vi "GetGyroAngle.vi"(8 "error in":errorcluster) -> (0 "error out":errorcluster, 3 "Angle":dbl)   [LabVIEW 2016]
uses:
  Robot Global Data.vi
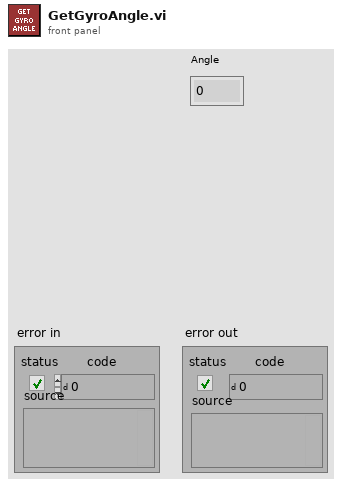
[diagram p1: front panel]
types:
  T1 = cluster{"Yaw":dbl, "Roll":dbl, "Pitch":dbl, "Heading":dbl, "Fused Heading":dbl}
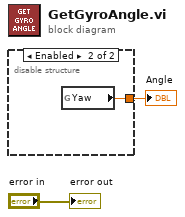
[diagram p0: block diagram]
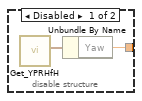
[diagram p2: hidden frame]
diagram:
  n1 = disable-structure shown="Enabled" {
    disable-tunnel: [w3 w5] -> w1
    frame Disabled {
      n2 = call <vilib>:"Get_YPRHfH.vi"() -> ("YRPHfH"=w4:T1)  [unwired: 11 in]
      n3 = Unbundle By Name(w4) -> ("Yaw"=w3:dbl)
    }
    frame Enabled {
      n4 = global read "Robot Global Data.vi" "Yaw"() -> (w5:dbl)
    }
  }
  "Angle" <- w1
  "error out" <- "error in"
